vi "5.4.vi"() -> ()   [LabVIEW 2017]
uses:
  <vilib>/measure/NI_MABase.lvlib
panel:
  out "波形图":waveform(dbl)(graph)
  in  "相位":dbl format="%.2p"
  in  "频率":dbl=10.0 format="%0.2p"
  in  "幅值":dbl=1.0 format="%0.2p"
  in  "sampling info":cluster{"Fs":dbl, "#s":dbl}={"Fs"=1000.0, "#s"=1000.0} caption="采样信息" {"Fs" format="%.2p"}
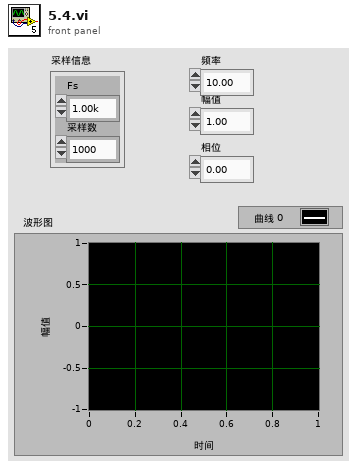
[diagram p1: front panel]
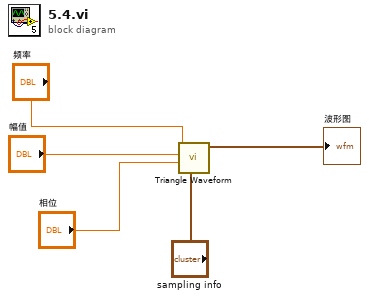
[diagram p0: block diagram]
diagram:
  n1 = call <vilib>:"Triangle Waveform.vi"("sampling info"="sampling info", "phase"="相位", "amplitude"="幅值", "frequency"="频率") -> ("signal out"=→"波形图":waveform(dbl))  [unwired: 6 in, 1 out]
